vi "Connect Sensor.vi"(8 "error in (no error)":errorcluster, 9 "lpszDataPath":string, 10 "nSensorIP":u32, 11 "nHostIP":u32) -> (0 "error out":errorcluster, 1 "lpszDataPath out":string, 3 "function return":i32)   [LabVIEW 2017, in "imgAcquisiotn.lvlib"]
doc: "DLLFunction int __stdcall ImageCapConnectSensor(unsigned int nHostIP, unsigned int nSensorIP, LPCTSTR lpszDataPath);"
uses:
  imgAcquisiotn.lvlib
  lib/ImageCaptureDLL.dll
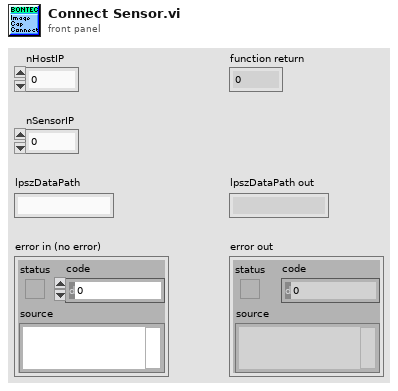
[diagram p1: front panel]
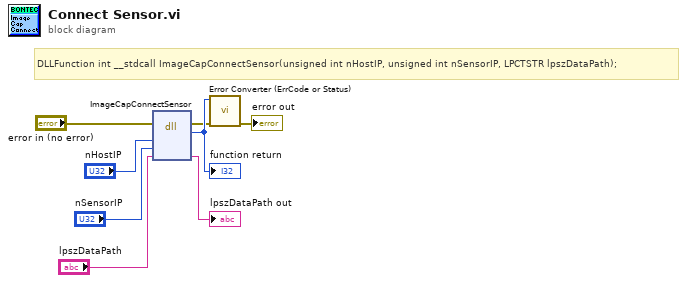
[diagram p0: block diagram]
diagram:
  # "DLLFunction int __stdcall ImageCapConnectSensor(unsigned int nHostIP, unsigned int nSensorIP, LPCTSTR lpszDataPath);"
  n1 = dll-call lib="F:/BonTechFlatPanelLVDriver/lib/ImageCaptureDLL.*" fn="ImageCapConnectSensor"(error in="error in (no error)", "nHostIP"="nHostIP", "nSensorIP"="nSensorIP", "lpszDataPath"="lpszDataPath") -> (error out=w2:errorcluster, w8:i32, "lpszDataPath"=→"lpszDataPath out":string)  [unwired: 4 in, 1 out]
  "function return" <- w8
  n2 = call "Error Converter (ErrCode or Status).vi"("error in (no error)"=w2, "error code"=w8) -> ("error out"=→"error out":errorcluster)  [unwired: 9 in]
